vi "Get Connection Information.vi"() -> ()   [LabVIEW 2018]
uses:
  TwinCAT ADS Class/Controls/Connection Information.ctl
  TwinCAT ADS Class/Controls/Address.ctl
  TwinCAT ADS Class/Controls/Connection Protocol.ctl
  TwinCAT ADS Class/Controls/Router State.ctl
  TwinCAT ADS Class/Controls/Connection State.ctl
  TwinCAT ADS Class/TwinCAT ADS.lvclass
panel:
  out "Connection Information":T1
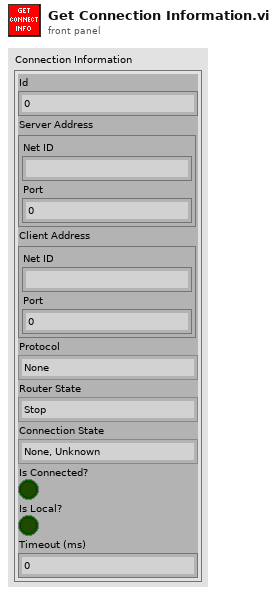
[diagram p1: front panel]
types:
  T1 = typedef "TwinCAT ADS.lvclass/Connection Information.ctl" = cluster{"Id":i32, "Server Address":T2, "Client Address":cluster{"Net ID":string, "Port":i32}, "Protocol":T3, "Router State":T4, "Connection State":T5, "Is Connected?":bool, "Is Local?":bool, "Timeout (ms)":i32}
  T2 = typedef "TwinCAT ADS.lvclass/Address.ctl" = cluster{"Net ID":string, "Port":i32}
  T3 = typedef "TwinCAT ADS.lvclass/Connection Protocol.ctl" = enum16{"None", "Router", "TCP/IP", "All"}
  T4 = typedef "TwinCAT ADS.lvclass/Router State.ctl" = enum16{"Stop", "Start", "Removed", "Unknown"}
  T5 = typedef "TwinCAT ADS.lvclass/Connection State.ctl" = enum16{"None, Unknown", "Disconnected", "Connected", "Lost"}
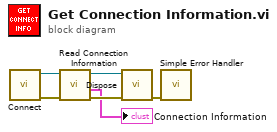
[diagram p0: block diagram]
diagram:
  n1 = call "Connect.vi"() -> ("error out"=w5:errorcluster, "TwinCAT ADS out"=w6:refnum<class "TwinCAT ADS.lvclass">)  [unwired: 10 in]
  n2 = call "Read Connection Information.vi"("error in (no error)"=w5, "TwinCAT ADS in"=w6) -> ("error out"=w2:errorcluster, "Connection Information"=→"Connection Information":T1, "TwinCAT ADS out"=w3:refnum<class "TwinCAT ADS.lvclass">)  [unwired: 7 in]
  n3 = call "Dispose.vi"("error in (no error)"=w2, "TwinCAT ADS in"=w3) -> ("error out"=w4:errorcluster)  [unwired: 9 in]
  n4 = call <vilib>:"Simple Error Handler.vi"("error in (no error)"=w4) -> ()  [unwired: 4 in, 5 out]
